vi "add_center_and_units.vi"(0 "TrajectoryTS090820Circular2D in":refnum<class "TrajectoryTS090820Circular2D.lvclass">, 5 "x trajectory":dbl[](array[numeric]), 7 "y trajectory":dbl[](array[numeric]), 9 "z trajectory":dbl[](array[numeric]), 11 "error in (no error)":errorcluster) -> (4 "TrajectoryTS090820Circular2D out":refnum<class "TrajectoryTS090820Circular2D.lvclass">, 6 "x centered trajectory":dbl[unit][](array[numeric]), 8 "y centered trajectory":dbl[unit][](array[numeric]), 10 "z centered trajectory":dbl[unit][](array[numeric]), 15 "error out":errorcluster)   [LabVIEW 2010, in "TrajectoryTS090820Circular2D.lvclass"]
uses:
  TrajectoryTS090820Circular2D.lvclass
  <vilib>/Analysis/NI_AALPro.lvlib
  <vilib>/Analysis/coordinate.llb/2D Cartesian Coordinate Rotation (Array).vi
  <vilib>/express/express arith-compare/Formula/XNode/ExpressFormulaBlockNode.xnode
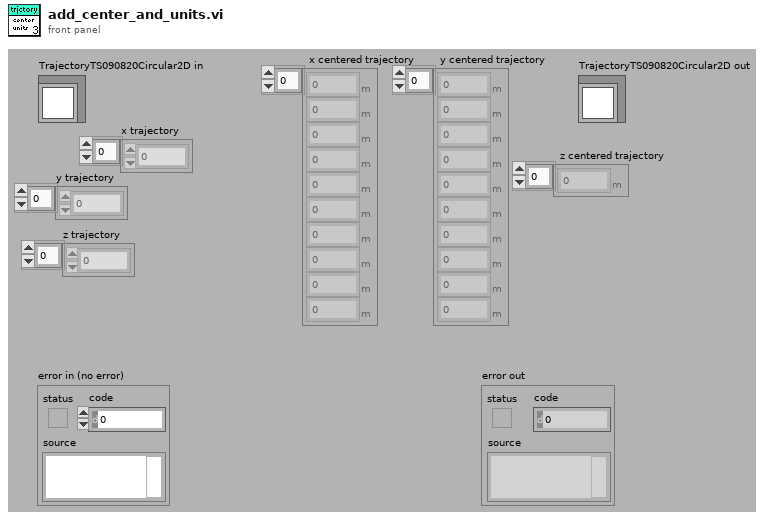
[diagram p1: front panel]
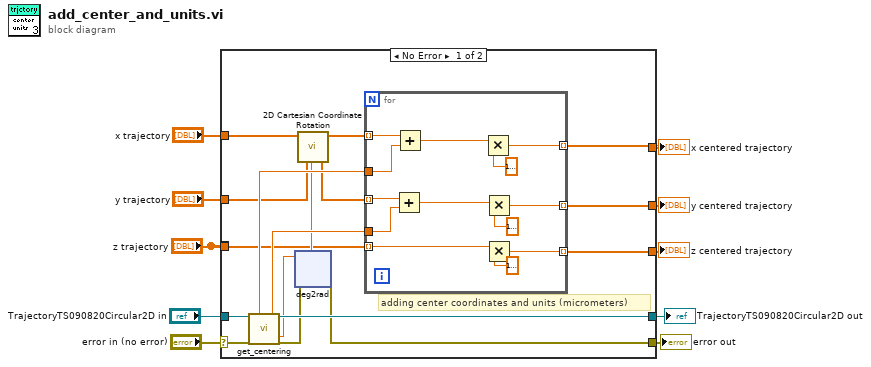
[diagram p0: block diagram]
diagram:
  n1 = case shown="No Error" "error in (no error)" {
    selector: "error in (no error)" -> [w27 w50]
    tunnel: [w13 w50] -> w9
    tunnel: [w25 w49] -> w7
    tunnel: "TrajectoryTS090820Circular2D in" -> [w26 w49]
    tunnel: "x trajectory" -> [w20 _]
    tunnel: "y trajectory" -> [w18 _]
    tunnel: [w22 _] -> w4
    tunnel: [w21 _] -> w3
    tunnel: "z trajectory" -> [_ _]
    tunnel: "z trajectory" -> [w12 _]
    tunnel: [w11 _] -> w1
    frame No Error {
      # "adding center coordinates and units (micrometers)"
      n2 = call-dynamic "get_centering.vi"("TrajectoryTS090820Circular2D in"=w26, "error in (no error)"=w27) -> ("TrajectoryTS090820Circular2D out"=w25:refnum<class "TrajectoryTS090820Circular2D.lvclass">, "x center"=w24:dbl, "y center"=w23:dbl, "rotation angle"=w16:dbl, "error out"=w14:errorcluster)  [unwired: 12 in, 1 out]
      n3 = xnode "deg2rad"("Xdeg"=w16, "error in (no error)"=w14) -> ("Result"=w15:dbl, "error out"=w13:errorcluster)
      n4 = call-poly <vilib>:"2D Cartesian Coordinate Rotation.vi"("theta"=w15, "Y"=w18, "X"=w20) -> ("Y Out"=w17:dbl[], "X Out"=w19:dbl[])  [unwired: 6 in, 1 out]
      n5 = for {
        tunnel: w19 -> [w46] mode=indexing
        tunnel: w17 -> [w45] mode=indexing
        tunnel: w24 -> [w37]
        tunnel: w23 -> [w36]
        tunnel: [w42] -> w22 mode=indexing
        tunnel: [w41] -> w21 mode=indexing
        tunnel: w12 -> [w39] mode=indexing
        tunnel: [w38] -> w11 mode=indexing
        n6 = Add(x=w45, y=w36) -> (x+y=w43:dbl)
        n7 = Add(x=w46, y=w37) -> (x+y=w44:dbl)
        n8 = Multiply(x=w44, y=dbl[unit] 1e-06 ("dimension size")) -> (x*y=w42:dbl[unit])
        n9 = Multiply(x=w43, y=dbl[unit] 1e-06 ("dimension size")) -> (x*y=w41:dbl[unit])
        n10 = Multiply(x=w39, y=dbl[unit] 1e-06 ("dimension size")) -> (x*y=w38:dbl[unit])
      }
    }
    frame Error {
    }
  }
  "error out" <- w9
  "TrajectoryTS090820Circular2D out" <- w7
  "x centered trajectory" <- w4
  "y centered trajectory" <- w3
  "z centered trajectory" <- w1
